vi "setUp.vi"(8 "error in (no error)":errorcluster, 11 "reference in":refnum<class "Test sqlite3.lvclass">) -> (0 "error out":errorcluster, 3 "reference out":refnum<class "Test sqlite3.lvclass">)   [LabVIEW 2020, in "Test sqlite3.lvclass"]
doc: "setUp runs prior to the test method during test execution. Use this method to initialize any object data required by your tests."
uses:
  Test sqlite3.lvclass
  <vilib>/addons/_JKI Toolkits/VI Tester/TestCase.llb/TestCase.lvclass
  Source/sqlite3/Source/sqlite3.lvclass
  C:/Program Files/National Instruments/LabVIEW 2020/vi.lib/addons/_JKI Toolkits/VI Tester/TestCase.llb/TestCase.lvclass
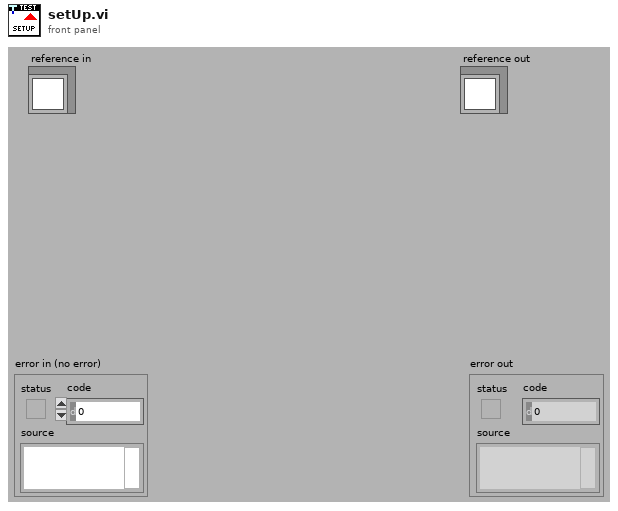
[diagram p1: front panel]
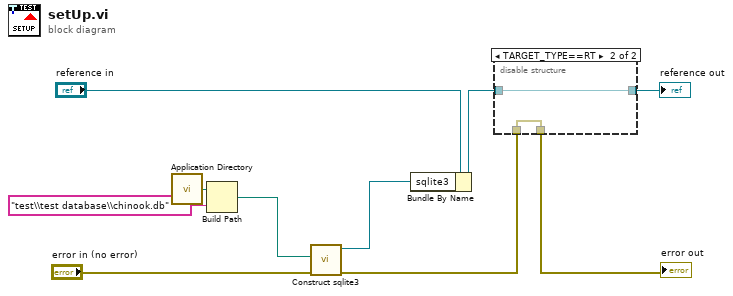
[diagram p0: block diagram]
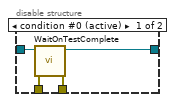
[diagram p2: hidden frame]
diagram:
  n1 = call <vilib>:"Application Directory.vi"() -> ("Application Directory"=w3:path)
  n2 = Build Path(base path=w3, name or relative path="test\\test database\\chinook.db") -> (appended path=w4:path)
  n3 = call "Construct sqlite3.vi"("error in (no error)"="error in (no error)", "DatabaseFilePath"=w4) -> ("error out"=w5:errorcluster, "sqlite3 out"=w1:refnum<class "sqlite3.lvclass">)  [unwired: 8 in]
  n4 = Bundle By Name(cluster="reference in", "sqlite3"=w1) -> (w7:refnum<class "Test sqlite3.lvclass">)
  n5 = disable-structure shown="TARGET_TYPE==RT" {
    disable-tunnel: w5 -> [w14 w15]
    disable-tunnel: [w13 w15] -> w10
    disable-tunnel: [w12 w16] -> w8
    disable-tunnel: w7 -> [w11 w16]
    frame condition #0 (active) {
      n6 = call <vilib>:"WaitOnTestComplete.vi"("error in (no error)"=w14, "TestCase in"=w11) -> ("error out"=w13:errorcluster, "TestCase out"=w12:refnum<class "Test sqlite3.lvclass">)  [unwired: 8 in]
    }
    frame condition #1 {
    }
  }
  "error out" <- w10
  "reference out" <- w8
